vi "host_wifi.vi"() -> ()   [LabVIEW 2019]
doc: "The Clap Sensor sample project implements a clap sensor that detects claps and displays the intensity of the claps by using the onboard LEDs of myRIO."
uses:
  <vilib>/myRIO/Instrument Drivers/Onboard IO/AI/typedefs/AI Reference.ctl
  <vilib>/myRIO/Common/Instrument Driver Framework/Utilities/typedefs/myRIO Generic Hardware Reference.ctl
  <vilib>/myRIO/Common/Instrument Driver Framework/Utilities/typedefs/Hardware Version Enum.ctl
  <vilib>/myRIO/Common/Instrument Driver Framework/Utilities/typedefs/myRIO v1.0 Reference.ctl
  <vilib>/myRIO/Common/Instrument Driver Framework/Utilities/typedefs/Generic FPGA Reference.ctl
  <vilib>/myRIO/Common/Instrument Driver Framework/myRIO v1.0/AI/typedefs/AI Channels List.ctl
  <vilib>/myRIO/Common/Instrument Driver Framework/myRIO v1.0/AI/typedefs/AI Channels Enum.ctl
  <vilib>/myRIO/Common/Instrument Driver Framework/Utilities/typedefs/Analog Scaling Constants List.ctl
  <vilib>/myRIO/Common/Instrument Driver Framework/Utilities/typedefs/Analog Scaling Constants.ctl
  <vilib>/userDefined/High Color/nirio_resource_hc.ctl
  <vilib>/myRIO/Instrument Drivers/Onboard IO/DIO/typedefs/DIO Reference.ctl
  <vilib>/myRIO/Common/Instrument Driver Framework/myRIO v1.0/DIO/typedefs/DIO Channels List.ctl
  <vilib>/myRIO/Common/Instrument Driver Framework/myRIO v1.0/DIO/typedefs/DIO Channels Enum.ctl
  <vilib>/Platform/TimedLoop/XDataNode/timing_clust.ctl
  <vilib>/Platform/TimedLoop/XDataNode/nitl_modes.ctl
  <vilib>/Platform/TimedLoop/XDataNode/wakeup.ctl
  <vilib>/myRIO/Common/Instrument Driver Framework/myRIO v1.0/AI/vis/myRIO v1.1 Open AI.vi
  <vilib>/myRIO/Common/Instrument Driver Framework/Utilities/vis/Is FPGA Ref Available.vi
  <vilib>/myRIO/Common/Instrument Driver Framework/myRIO v1.0/DIO/vis/myRIO v1.1 Open DIO.vi
  <vilib>/myRIO/Common/Instrument Driver Framework/Utilities/vis/Validate Channels.vi
  <vilib>/myRIO/Common/Instrument Driver Framework/myRIO v1.0/AI/vis/myRIO v1.0 Reserve AI.vi
  <vilib>/myRIO/Common/Instrument Driver Framework/myRIO v1.0/DIO/vis/myRIO v1.0 Reserve DIO.vi
  <vilib>/myRIO/Common/Instrument Driver Framework/myRIO v1.0/UART/vis/myRIO v1.0 Close UART.vi
  <vilib>/myRIO/Common/Instrument Driver Framework/myRIO v1.0/AI/vis/myRIO v1.0 Build MUX Configuration AI.vi
  <vilib>/myRIO/Common/Instrument Driver Framework/myRIO v1.0/Resource Manager/vis/myRIO v1.0 Reserve Channel List.vi
  <vilib>/myRIO/Common/Instrument Driver Framework/myRIO v1.0/DIO/vis/myRIO v1.0 Build MUX Configuration DIO.vi
  <vilib>/myRIO/Common/Instrument Driver Framework/myRIO v1.0/Resource Manager/vis/myRIO v1.0 Reserve Channel.vi
  <vilib>/myRIO/Common/Instrument Driver Framework/myRIO v1.0/Resource Manager/vis/myRIO v1.0 Unreserve Channel.vi
  <vilib>/myRIO/Common/Instrument Driver Framework/myRIO v1.0/Resource Manager/vis/myRIO v1.0 Create Configuration List.vi
  <vilib>/myRIO/Common/Instrument Driver Framework/myRIO v1.0/Resource Manager/vis/myRIO v1.0 Build Mutex Name.vi
  <vilib>/Utility/VariantDataType/GetNumericInfo.vi
  <vilib>/Utility/error.llb/Error Cluster From Error Code.vi
  <vilib>/myRIO/Common/Instrument Driver Framework/myRIO v1.0/myRIO v1.1 Open.vi
  <vilib>/myRIO/Common/Instrument Driver Framework/myRIO v1.0/AI/vis/myRIO v1.0 Get Scaling Constants AI.vi
  <vilib>/myRIO/Common/Instrument Driver Framework/Utilities/vis/IO Manager.vi
  <vilib>/myRIO/Common/Instrument Driver Framework/Utilities/vis/Configuration Manager.vi
  <vilib>/myRIO/Common/Instrument Driver Framework/myRIO v1.0/myRIO v1.0 Close.vi
  <vilib>/myRIO/Common/Instrument Driver Framework/myRIO v1.0/Resource Manager/vis/myRIO v1.0 Configure IO.vi
  <vilib>/myRIO/Common/Instrument Driver Framework/myRIO v1.0/DIO/vis/myRIO v1.0 Read DIO.vi
  <vilib>/myRIO/Common/Instrument Driver Framework/myRIO v1.0/AI/vis/myRIO v1.0 Read AI.vi
  <vilib>/myRIO/Common/Instrument Driver Framework/myRIO v1.0/DIO/vis/myRIO v1.0 Write DIO.vi
  <vilib>/myRIO/Instrument Drivers/Onboard IO/DIO/vis/Smart Open.vi
  <vilib>/myRIO/Common/Instrument Driver Framework/Utilities/vis/FPGA Ref Manager.vi
  <vilib>/myRIO/Common/Instrument Driver Framework/myRIO v1.0/myRIO v1.0 Reset FPGA.vi
  <vilib>/myRIO/Common/Instrument Driver Framework/myRIO v1.0/IRQ/vis/myRIO v1.0 IRQ Info FGV.vi
  <vilib>/myRIO/Common/Instrument Driver Framework/myRIO v1.0/IRQ/vis/myRIO v1.0 Timer IRQ Info FGV.vi
  <vilib>/myRIO/Common/Instrument Driver Framework/myRIO v1.0/IRQ/vis/myRIO v1.0 ISR Agent.vi
  <vilib>/myRIO/Instrument Drivers/Utilities/vis/Reset Index.vi
  <vilib>/myRIO/Common/Instrument Driver Framework/myRIO v1.0/Resource Manager/vis/myRIO v1.0 Block Write Resource Manager.vi
  <vilib>/myRIO/Instrument Drivers/Onboard IO/AI/vis/myRIO AI Open.xnode
  <vilib>/myRIO/Express VI/Onboard Devices/Button/Button Express VI.xnode
  <vilib>/myRIO/Instrument Drivers/Onboard IO/DIO/vis/myRIO DIO Open.xnode
  <vilib>/Platform/TimedLoop/XDataNode/XDataNode.xnode
  <vilib>/myRIO/Instrument Drivers/Onboard IO/AI/AI.lvlib
  <vilib>/myRIO/Instrument Drivers/Onboard IO/DIO/DIO.lvlib
  <vilib>/myRIO/Instrument Drivers/Utilities/Utilities.lvlib
  <vilib>/Platform/TimedLoop/XDataNode/XDNodeRunTimeDep.lvlib
panel:
  out "freq_send":dbl
  out "key_pressed(n)":dbl
  in  "stop_playing":bool
  out "Keypad buttons":bool[][](array[boolean])
  in  "stop_recording":bool
  # "Overview: The Clap Sensor sample project implements a clap sensor that detects claps and displays the intensity of the claps by using the onboard LEDs of myRIO.\nInstructions:\n1. Connect a microphone to the audio input jack.\n2. Run this VI"
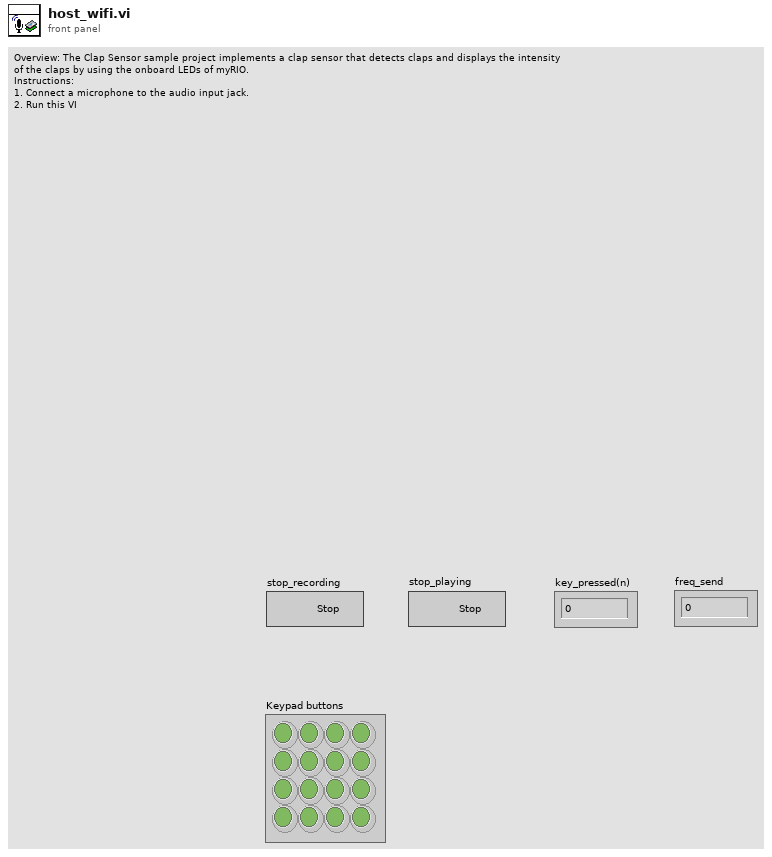
[diagram p1: front panel]
types:
  T1 = typedef "nirio_resource_hc.ctl" = tag
  T2 = typedef "Hardware Version Enum.ctl" = enum16{"Unknown", "myRIO-1900", "myRIO-1950", "roboRIO", "NI ELVIS RIO CM", "ELVIS III"}
  T3 = typedef "XDNodeRunTimeDep.lvlib/timing_clust.ctl" = cluster{"Expected End [f-1]":u64, "Actual End [f-1]":u64, "Finished Late? [f-1]":bool, "Expected End [i-1]":u64, "Actual End [i-1]":u64, "Finished Late? [i-1]":bool, "Expected Start [i]":u64, "Actual Start [i]":u64, "Expected Start [f]":u64, "Actual Start [f]":u64, "Source Name":string, "Structure Name":string, "Period":i64, "Deadline":i64, "Offset":i64, "Start":i64, "Priority":i32, "Timeout":i32, "Mode":T4, "Wakeup Reason":T5, "Error":errorcluster, "Source Type":string, "Secondary Source Type":string, "Global End Time":u64, "Global Start Time":u64, "Frame Duration":u64, "Iteration Duration":u64, "Assigned CPU":i32, "I/O Scan Engine Mode":u32}
  T4 = typedef "XDNodeRunTimeDep.lvlib/nitl_modes.ctl" = enum32{"No Change", "Process missed periods, maintain original phase", "Discard missed periods, maintain original phase", "Process missed periods, ignore original phase", "Discard missed periods, ignore original phase"}
  T5 = typedef "XDNodeRunTimeDep.lvlib/wakeup.ctl" = enum32{"Normal", "Aborted", "Asynchronous wakeup", "Timing source error", "Timed loop error", "Timeout"}
  T6 = typedef "DIO.lvlib/DIO Reference.ctl" = cluster{"myRIO Reference":T7, "DIO Channels List":T10}
  T7 = typedef "myRIO Generic Hardware Reference.ctl" = cluster{"myRIO Model":T2, "myRIO Hardware Reference":T8}
  T8 = typedef "myRIO v1.0 Reference.ctl" = cluster{"Generic FPGA Reference":T9, "Allow multiple opens":bool}
  T9 = typedef "Generic FPGA Reference.ctl" = refnum<k20>
  T10 = typedef "DIO Channels List.ctl" = T11[]
  T11 = typedef "DIO Channels Enum.ctl" = enum16{"Not Connected", "C/DIO0", "C/DIO1", "C/DIO2", "C/DIO3", "C/DIO4", "C/DIO5", "C/DIO6", "C/DIO7", "A/DIO0", "A/DIO1", "A/DIO2", "A/DIO3", "A/DIO4", "A/DIO5", "A/DIO6", "A/DIO7", "A/DIO8", "A/DIO9", "A/DIO10", "A/DIO11", "A/DIO12", "A/DIO13", "A/DIO14", "A/DIO15", "A/DIO16", "A/DIO17", "A/DIO18", "A/DIO19", "B/DIO0", "B/DIO1", "B/DIO2", "B/DIO3", "B/DIO4", "B/DIO5", "B/DIO6", "B/DIO7", "B/DIO8", "B/DIO9", "B/DIO10", "B/DIO11", "B/DIO12", "B/DIO13", "B/DIO14", "B/DIO15", "B/DIO16", "B/DIO17", "B/DIO18", "B/DIO19", "LED0", "LED1", "LED2", "LED3", "Button0", "DIO/DIO0", "DIO/DIO1", "DIO/DIO2", "DIO/DIO3", "DIO/DIO4", "DIO/DIO5", "DIO/DIO6", "DIO/DIO7", "DIO/DIO8", "DIO/DIO9", "SPI/CS0", "SPI/CS1", "SPI/CS2", "SPI/CS3", "LED RADIO (Green)", "LED RADIO (Red)", "LED COMM (Green)", "LED COMM (Red)", "LED MODE (Green)", "LED MODE (Red)"}
  T12 = typedef "AI.lvlib/AI Reference.ctl" = cluster{"myRIO Reference":T7, "AI Channels List":T13, "AI Scaling Constants List":T15}
  T13 = typedef "AI Channels List.ctl" = T14[]
  T14 = typedef "AI Channels Enum.ctl" = enum16{"Not Connected", "AudioIn/Left", "AudioIn/Right", "C/AI0", "C/AI1", "A/AI0", "A/AI1", "A/AI2", "A/AI3", "A/AI4", "A/AI5", "A/AI6", "A/AI7", "B/AI0", "B/AI1", "B/AI2", "B/AI3", "B/AI4", "B/AI5", "B/AI6", "B/AI7", "AI/AI0", "AI/AI1", "AI/AI2", "AI/AI3", "A/AI0 (DIFF)", "A/AI1 (DIFF)", "A/AI2 (DIFF)", "A/AI3 (DIFF)", "B/AI0 (DIFF)", "B/AI1 (DIFF)", "B/AI2 (DIFF)", "B/AI3 (DIFF)"}
  T15 = typedef "Analog Scaling Constants List.ctl" = T16[]
  T16 = typedef "Analog Scaling Constants.ctl" = cluster{"LSB Weight (Volts)":dbl, "Offset (Volts)":dbl, "Signed?":bool}
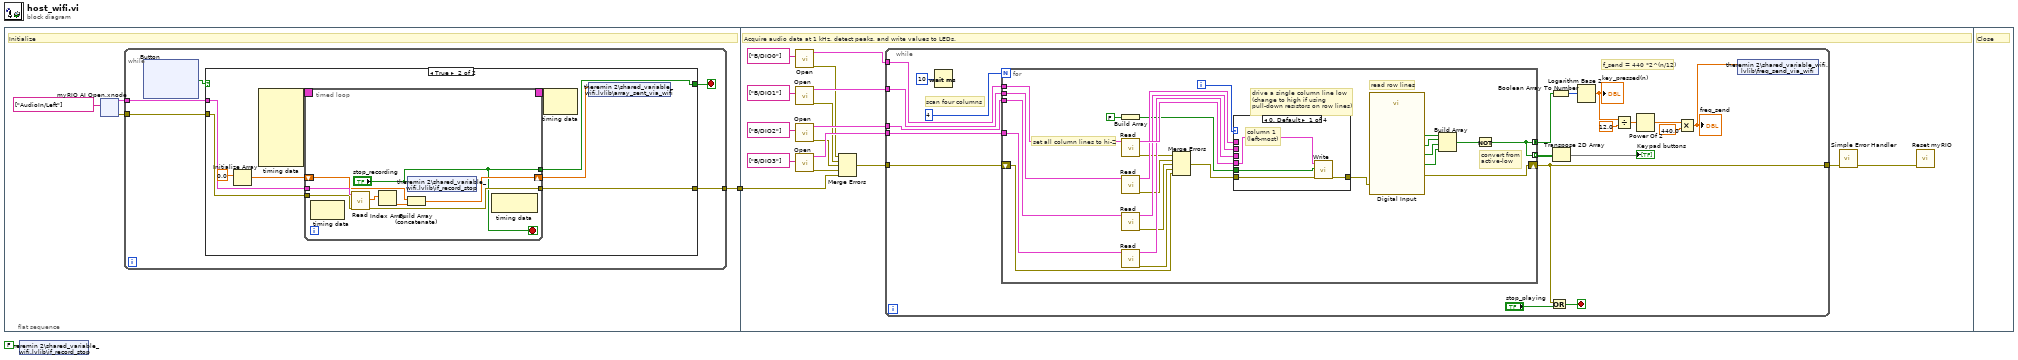
[diagram p0: block diagram]
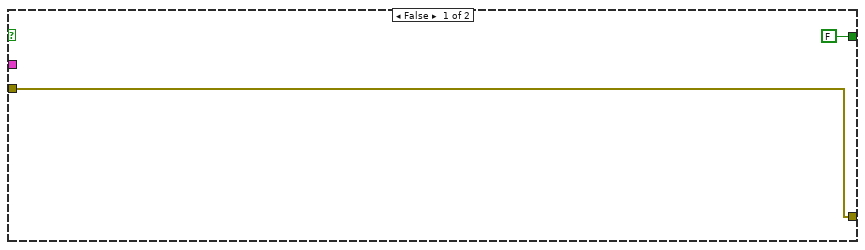
[diagram p2: hidden frame]
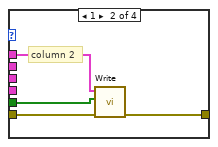
[diagram p3: hidden frame]
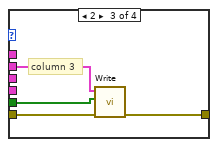
[diagram p4: hidden frame]
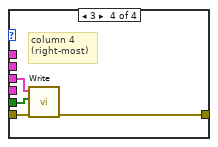
[diagram p5: hidden frame]
diagram:
  n1 = flat-sequence {
    tunnel: [w3] -> w2
    tunnel: w2 -> [w88]
    frame #0 {
      # "Initialize"
      n2 = xnode "myRIO AI Open.xnode"("Channel Names"=tag[] ["AudioIn/Left"]) -> ("error out"=w5:errorcluster, "AI Ref Out"=w4:T12)  [unwired: 2 in]
      n3 = while {
        tunnel: w5 -> [w29]
        tunnel: w4 -> [w28]
        tunnel: [w25] -> w3
        stop <- w27 stop-if-true
        n4 = xnode "Button"() -> ("Value"=w26:bool)  [unwired: 1 in, 1 out]
        n5 = case shown="True" w26 {
          tunnel: w29 -> [w30 w40]
          tunnel: w28 -> [_ w39]
          tunnel: [FALSE ("Stop Button") w38] -> w27
          tunnel: [w30 w35] -> w25
          frame False {
          }
          frame True {
            n6 = Initialize Array(0.0 ("element")) -> (w37:dbl[])  [unwired: 1 in]
            n7 = node-c288() -> (w34:T3)  [unwired: 7 in]
            n8 = timed-loop {
              tunnel: w39 -> [w48]
              tunnel: w40 -> [w47]
              tunnel: ["stop_recording"] -> w38
              shift-right: [w46] -> w32
              shift-left: w37 -> [w45]
              tunnel: [w43] -> w35
              timing: w34 -> [_]
              timing-out: [_] -> w33
              stop <- "stop_recording" stop-if-true
              n9 = node-c288() -> ()  [unwired: 1 in, 1 out]
              n10 = call <vilib>:"Read.vi"("error in (no error)"=w47, "AI Ref In"=w48) -> ("error out"=w43:errorcluster, "Values"=w42:dbl[])  [unwired: 7 in, 1 out]
              n11 = Index Array(array=w42) -> (element=w44:dbl)  [unwired: 1 in]
              n12 = shared-variable "theremin 2\\shared_variable_wifi.lvlib\\if_record_stop"("stop_recording") -> ()  [unwired: 1 in, 1 out]
              n13 = Build Array (concatenate)(w45, w44) -> (w46:dbl[])
              n14 = node-c288() -> ()  [unwired: 1 in, 1 out]
            }
            n15 = node-c288(w33) -> ()  [unwired: 1 out]
            n16 = shared-variable "theremin 2\\shared_variable_wifi.lvlib\\array_sent_via_wifi"(w32) -> ()  [unwired: 1 in, 1 out]
          }
        }
      }
    }
    frame #1 {
      # "Acquire audio data at 1 kHz, detect peaks, and write values to LEDs."
      n17 = call <vilib>:"Open.vi"("Channel Names"=tag[] ["B/DIO0"]) -> ("error out"=w93:errorcluster, "DIO Ref Out"=w97:T6)  [unwired: 9 in]
      n18 = call <vilib>:"Open.vi"("Channel Names"=tag[] ["B/DIO1"]) -> ("error out"=w92:errorcluster, "DIO Ref Out"=w96:T6)  [unwired: 9 in]
      n19 = call <vilib>:"Open.vi"("Channel Names"=tag[] ["B/DIO2"]) -> ("error out"=w91:errorcluster, "DIO Ref Out"=w95:T6)  [unwired: 9 in]
      n20 = call <vilib>:"Open.vi"("Channel Names"=tag[] ["B/DIO3"]) -> ("error out"=w90:errorcluster, "DIO Ref Out"=w94:T6)  [unwired: 9 in]
      n21 = Merge Errors "Merge Errors"(w93, w92, w91, w90, w88) -> (w89:errorcluster)
      n22 = while {
        tunnel: [w119] -> w103
        tunnel: w97 -> [w116]
        tunnel: w96 -> [w115]
        tunnel: w95 -> [w114]
        tunnel: w94 -> [w113]
        tunnel: w89 -> [w112]
        stop <- w123 stop-if-true
        # "f_send = 440 *2^(n/12)"
        # "scan four columns"
        n23 = Wait (ms)(milliseconds to wait=u32 10) -> ()  [unwired: 1 out]
        n24 = for {
          N: 4 -> [_]
          tunnel: [w141] -> w118 mode=indexing
          shift-right: [w143] -> w119
          shift-left: w112 -> [w127]
          tunnel: [w141] -> w105 mode=concatenating
          tunnel: w116 -> [w140]
          tunnel: w115 -> [w137]
          tunnel: w114 -> [w138]
          tunnel: w113 -> [w139]
          i -> [w148]
          # "convert from\nactive-low"
          # "set all column lines to hi-Z"
          # "read row lines"
          # "drive a single column line low\n(change to high if using \npull-down resistors on row lines)"
          n25 = Build Array "Build Array"(FALSE) -> (w124:bool[])
          n26 = call <vilib>:"Read.vi"("DIO Ref In"=w140) -> ("error out"=w131:errorcluster, "DIO Ref Out"=w136:T6)  [unwired: 8 in, 1 out]
          n27 = call <vilib>:"Read.vi"("DIO Ref In"=w137) -> ("error out"=w130:errorcluster, "DIO Ref Out"=w135:T6)  [unwired: 8 in, 1 out]
          n28 = call <vilib>:"Read.vi"("DIO Ref In"=w138) -> ("error out"=w129:errorcluster, "DIO Ref Out"=w134:T6)  [unwired: 8 in, 1 out]
          n29 = call <vilib>:"Read.vi"("DIO Ref In"=w139) -> ("error out"=w128:errorcluster, "DIO Ref Out"=w133:T6)  [unwired: 8 in, 1 out]
          n30 = Merge Errors(w131, w130, w129, w128, w127) -> (w126:errorcluster)
          n31 = case shown="0, Default" w148 {
            tunnel: w136 -> [w152 _ _ _]
            tunnel: w135 -> [_ w156 _ _]
            tunnel: w134 -> [_ _ w160 _]
            tunnel: w133 -> [_ _ _ w164]
            tunnel: [w151 w155 w159 w163] -> w132
            tunnel: w126 -> [w150 w154 w158 w162]
            tunnel: w124 -> [w149 w153 w157 w161]
            frame 0, Default {
              # "column 1\n(left-most)"
              n32 = call <vilib>:"Write.vi"("error in (no error)"=w150, "Values"=w149, "DIO Ref In"=w152) -> ("error out"=w151:errorcluster)  [unwired: 6 in, 1 out]
            }
            frame 1 {
              # "column 2"
              n33 = call <vilib>:"Write.vi"("error in (no error)"=w154, "Values"=w153, "DIO Ref In"=w156) -> ("error out"=w155:errorcluster)  [unwired: 6 in, 1 out]
            }
            frame 2 {
              # "column 3"
              n34 = call <vilib>:"Write.vi"("error in (no error)"=w158, "Values"=w157, "DIO Ref In"=w160) -> ("error out"=w159:errorcluster)  [unwired: 6 in, 1 out]
            }
            frame 3 {
              # "column 4\n(right-most)"
              n35 = call <vilib>:"Write.vi"("error in (no error)"=w162, "Values"=w161, "DIO Ref In"=w164) -> ("error out"=w163:errorcluster)  [unwired: 6 in, 1 out]
            }
          }
          n36 = call "Digital Input"("error in (no error)"=w132) -> ("B/DIO4 (Pin 19)"=w147:bool, "B/DIO5 (Pin 21)"=w146:bool, "B/DIO6 (Pin 23)"=w145:bool, "B/DIO7 (Pin 25)"=w144:bool, "error out"=w143:errorcluster)  [unwired: 22 in]
          n37 = Build Array "Build Array"(w147, w146, w145, w144) -> (w142:bool[])
          n38 = Not(x=w142) -> (.not. x?=w141:bool[])
        }
        n39 = Or(x=w119, y="stop_playing") -> (x .or. y?=w123:bool)
        n40 = Boolean Array To Number(Boolean array=w105) -> (number=w111:u32)
        n41 = Transpose 2D Array(2D array=w118) -> (transposed array=→"Keypad buttons":bool[][])
        n42 = Logarithm Base 2(1:w111) -> (0:w110:dbl)
        "key_pressed(n)" <- w110
        n43 = Divide(x=w110, y=12.0) -> (x/y=w108:dbl)
        n44 = Power Of 2(x=w108) -> (2^x=w107:dbl)
        n45 = Multiply(x=w107, y=440.0) -> (x*y=w104:dbl)
        "freq_send" <- w104
        n46 = shared-variable "theremin 2\\shared_variable_wifi.lvlib\\freq_send_via_wifi"(w104) -> ()  [unwired: 1 in, 1 out]
      }
      n47 = call <vilib>:"Simple Error Handler.vi"("error in (no error)"=w103) -> ("error out"=w102:errorcluster)  [unwired: 4 in, 4 out]
      n48 = call <vilib>:"Reset myRIO.vi"("error in (no error)"=w102) -> ()  [unwired: 10 in, 1 out]
    }
    frame #2 {
      # "Close"
    }
  }
  n49 = shared-variable "theremin 2\\shared_variable_wifi.lvlib\\if_record_stop"(FALSE ("if_record_stop")) -> ()  [unwired: 1 in, 1 out]
